vi "6_3.vi"() -> ()   [LabVIEW 2017]
uses:
  <vilib>/measure/NI_MABase.lvlib
panel:
  out "Y":dbl[](array[numeric])
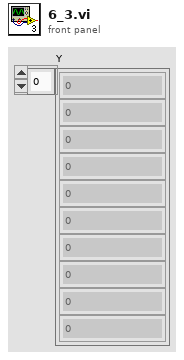
[diagram p1: front panel]
types:
  T1 = enum16{"open", "replace", "create", "open or create", "replace or create", "replace or create with confirmation"}
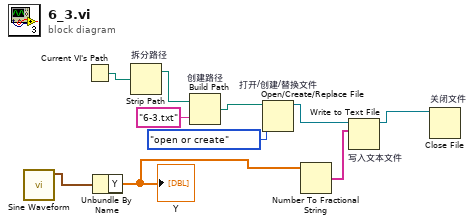
[diagram p0: block diagram]
diagram:
  n1 = call <vilib>:"Sine Waveform.vi"() -> ("signal out"=w10:waveform(dbl))  [unwired: 10 in, 1 out]
  n2 = Current VI's Path() -> (path=w2:path)
  n3 = Unbundle By Name(w10) -> ("Y"=w5:dbl[])
  "Y" <- w5
  n4 = Strip Path "拆分路径"(path=w2) -> (stripped path=w1:path)  [unwired: 1 out]
  n5 = Build Path "创建路径"(base path=w1, name or relative path="6-3.txt" ("名称或相对路径")) -> (appended path=w9:path)
  n6 = Open/Create/Replace File "打开/创建/替换文件"(file path (use dialog)=w9, operation (0:open)=T1."open or create" ("操作(0:open)")) -> (refnum out=w7:refnum<file>)  [unwired: 4 in, 2 out]
  n7 = Number To Fractional String(number=w5) -> (F-format string=w4:string[])  [unwired: 3 in]
  n8 = Write to Text File "写入文本文件"(file (use dialog)=w7, text=w4) -> (refnum out=w6:refnum<file>)  [unwired: 2 in, 2 out]
  n9 = Close File "关闭文件"(refnum=w6) -> ()  [unwired: 1 in, 2 out]
